vi "Pedestrian Signal Controller (configurable).vi"(8 "walk":bool, 11 "cars stopped":T1) -> (0 "ped signal":T2, 3 "peds stopped":T1)   [LabVIEW 2023]
uses:
  <extravilib>/ChannelInstances/One Element Stream-u16/)Channel.ctl
  <extravilib>/ChannelInstances/One Element Stream-bool/)Channel.ctl
  26a4a908-d1f9-ed44-88a4-6f9b1e837490.vi
  091f0f9f-ba83-5e49-bf52-7e477d967a4d.vi
  <extravilib>/ChannelInstances/One Element Stream-u16/Write With Abort.vi
  <extravilib>/ChannelInstances/One Element Stream-bool/Write With Abort.vi
  <extravilib>/ChannelInstances/One Element Stream-bool/Read With Abort.vi
  <extravilib>/ChannelInstances/One Element Stream-u16/Endpoint.vi
  <extravilib>/ChannelInstances/One Element Stream-bool/Endpoint.vi
  <extravilib>/ChannelInstances/One Element Stream-bool/EndpointRead.vi
  <extravilib>/ChannelInstances/One Element Stream-bool.lvlib
  <extravilib>/ChannelInstances/One Element Stream-u16.lvlib
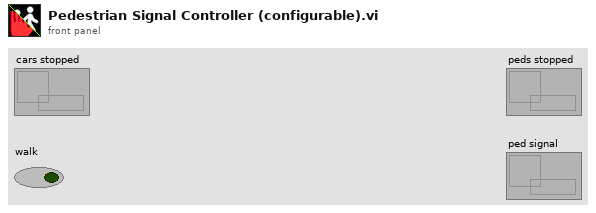
[diagram p1: front panel]
types:
  T1 = typedef "One Element Stream-bool.lvlib/)Channel.ctl" = refnum<queue>
  T2 = typedef "One Element Stream-u16.lvlib/)Channel.ctl" = refnum<queue>
  T3 = enum16{"_Quit_", "Wait", "Walk", "Flash", "Config"}
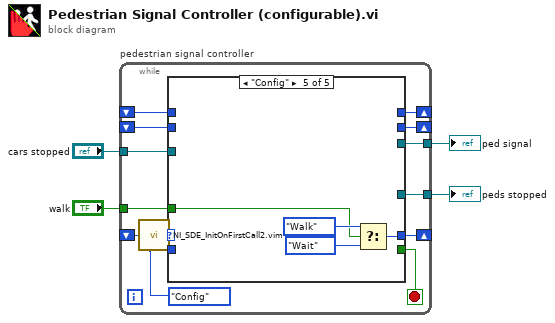
[diagram p0: block diagram]
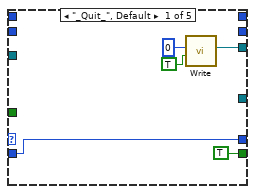
[diagram p2: hidden frame]
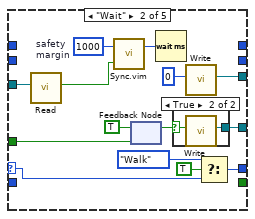
[diagram p3: hidden frame]
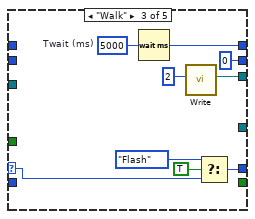
[diagram p5: hidden frame]
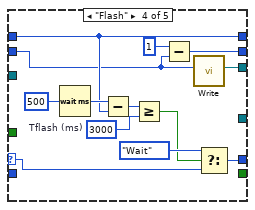
[diagram p6: hidden frame]
diagram:
  n1 = while "pedestrian signal controller" {
    tunnel: "cars stopped" -> [w16]
    shift-right: [w15] -> _
    shift-left: _ -> [w14]
    tunnel: [w13] -> w4
    shift-right: [w12] -> _
    shift-left: _ -> [w11]
    tunnel: [w10] -> w3
    tunnel: "walk" -> [w9]
    shift-right: [w7] -> _
    shift-left: _ -> [w6]
    stop <- w17 stop-if-true
    w8 = T3."Config"
    n2 = call "NI_SDE_InitOnFirstCall2.vim"("input"=w6, "master enum"=w8) -> ("output enum"=w5:T3)  [unwired: 1 in]
    n3 = case shown="\"Config\"" w5 {
      selector: w5 -> [_ w36 w47 w60 _]
      tunnel: [TRUE _ _ _ _] -> w17
      tunnel: [w18 w35 w46 w59 w64] -> w7
      tunnel: w16 -> [_ w33 _ _ _]
      tunnel: [_ _ w42 w53 _] -> w15
      tunnel: w14 -> [_ _ _ w53 _]
      tunnel: [w20 w31 w40 w52 _] -> w13
      tunnel: [_ _ u16 0 w50 _] -> w12
      tunnel: w11 -> [_ _ _ w49 _]
      tunnel: [_ w30 _ _ _] -> w10
      tunnel: w9 -> [_ w23 _ _ w61]
      tunnel: w8 -> [w18 _ _ _ _]
      frame "_Quit_", Default {
        n4 = call <extravilib>:"Write.vi"("last element? (F)"=TRUE, "element"=u16 0) -> ("channel"=w20:T2)  [unwired: 8 in, 1 out]
      }
      frame "Wait" {
        w27 = u32 1000  # safety margin
        n5 = call <extravilib>:"Read.vi"("channel"=w33) -> ("element"=w28:bool)  [unwired: 7 in, 3 out]
        n6 = call "Sync.vim"("a"=w27, "b"=w28) -> ("a'"=w26:u32)  [unwired: 24 in, 1 out]
        n7 = feedback-in #1(TRUE) -> ()
        n8 = feedback #1(w23) -> (w24:bool)
        n9 = Wait (ms)(milliseconds to wait=w26) -> ()  [unwired: 1 out]
        n10 = case shown="True" w24 {
          selector: w24 -> [_ w37]
          tunnel: [_ w38] -> w30
          frame False {
          }
          frame True {
            n11 = call <extravilib>:"Write.vi"("element"=w37) -> ("channel"=w38:T1)  [unwired: 9 in, 1 out]
          }
        }
        n12 = call <extravilib>:"Write.vi"("element"=u16 0) -> ("channel"=w31:T2)  [unwired: 9 in, 1 out]
        n13 = Select(t=T3."Walk", s=TRUE, f=w36) -> (s? t:f=w35:T3)
      }
      frame "Walk" {
        w44 = u32 5000  # Twait (ms)
        n14 = Wait (ms)(milliseconds to wait=w44) -> (millisecond timer value=w42:u32)
        n15 = call <extravilib>:"Write.vi"("element"=u16 2) -> ("channel"=w40:T2)  [unwired: 9 in, 1 out]
        n16 = Select(t=T3."Flash", s=TRUE, f=w47) -> (s? t:f=w46:T3)
      }
      frame "Flash" {
        w54 = u32 3000  # Tflash (ms)
        n17 = Wait (ms)(milliseconds to wait=u32 500) -> (millisecond timer value=w56:u32)
        n18 = Subtract(x=w56, y=w53) -> (x-y=w55:u32)
        n19 = Greater Or Equal?(x=w55, y=w54) -> (x >= y?=w48:bool)
        n20 = Subtract(x=u16 1, y=w49) -> (x-y=w50:u16)
        n21 = call <extravilib>:"Write.vi"("element"=w49) -> ("channel"=w52:T2)  [unwired: 9 in, 1 out]
        n22 = Select(t=T3."Wait", s=w48, f=w60) -> (s? t:f=w59:T3)
      }
      frame "Config" {
        n23 = Select(t=T3."Walk", s=w61, f=T3."Wait") -> (s? t:f=w64:T3)
      }
    }
  }
  "ped signal" <- w4
  "peds stopped" <- w3
